vi "YokoGS200 Get Output.vi"(0 "VISA Rsrc":refnum<visa-resource-name>="SR530", 3 "error in (no error)":errorcluster) -> (7 "VISA Rsrc Out":refnum<visa-resource-name>="GPIB0::12::INSTR", 8 "Output State":bool, 10 "error out":errorcluster)   [LabVIEW 2019]
panel:
  out "Octet d'état":bool[](array[boolean])
  out "octet d'état":u16
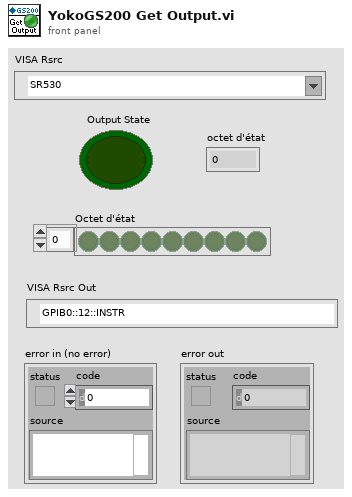
[diagram p1: front panel]
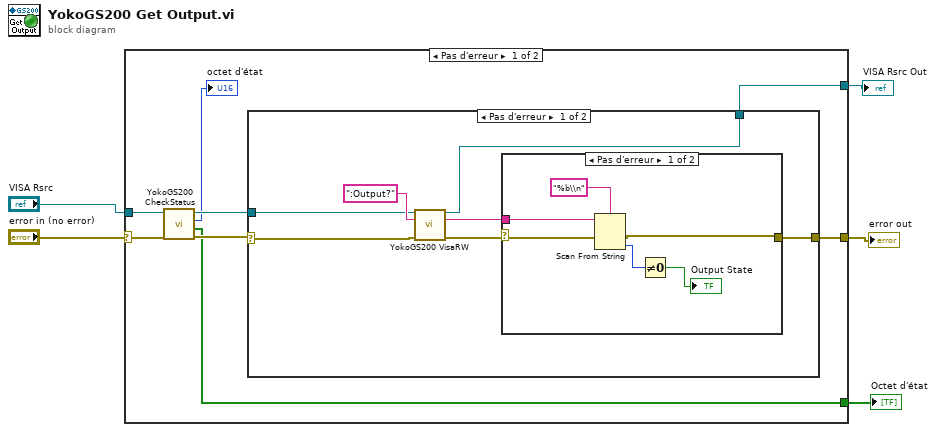
[diagram p0: block diagram]
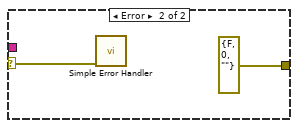
[diagram p2: hidden frame]
diagram:
  n1 = case shown="Pas d'erreur" "error in (no error)" {
    selector: "error in (no error)" -> [w12 w31]
    tunnel: "VISA Rsrc" -> [w11 w32]
    tunnel: [w13 w31] -> w3
    tunnel: [w8 w32] -> w2
    tunnel: [w7 _] -> w1
    frame No Error {
      n2 = call <userlib>:"YokoGS200 CheckStatus.vi"("error in (no error)"=w12, "VISA Rsrc"=w11) -> ("error out"=w10:errorcluster, "Octet d'état"=w7:bool[], "octet d'état"=→"octet d'état":u16, "VISA Rsrc Out"=w9:refnum<visa-resource-name>)  [unwired: 6 in]
      n3 = case shown="Pas d'erreur" w10 {
        selector: w10 -> [w16 w30]
        tunnel: [w19 w30] -> w13
        tunnel: w9 -> [w15 w29]
        tunnel: [w14 w29] -> w8
        frame No Error {
          n4 = call <userlib>:"YokoGS200 VisaRW.vi"("VISA Rsrc"=w15, "ChaineCom"=":Output?" ("initial string"), "error in (no error)"=w16) -> ("VISA Rsrc Out"=w14:refnum<visa-resource-name>, "ChaineRep"=w17:string, "error out"=w18:errorcluster)  [unwired: 8 in, 2 out]
          n5 = case shown="Pas d'erreur" w18 {
            selector: w18 -> [w26 w27]
            tunnel: [w23 errorcluster {"status"=FALSE, "code"=0, "source"=""} ("error IO")] -> w19
            tunnel: w17 -> [w25 _]
            frame No Error {
              n6 = Scan From String(format string="%b\\n", input string=w25, error in=w26) -> (error out=w23:errorcluster, output 1=w22:i32)  [unwired: 2 in, 2 out]
              n7 = Not Equal To 0?(x=w22) -> (x != 0?=→"Output State":bool)
            }
            frame Error {
              n8 = call <vilib>:"Simple Error Handler.vi"("error in (no error)"=w27) -> ()  [unwired: 4 in, 5 out]
            }
          }
        }
        frame Error {
        }
      }
    }
    frame Error {
    }
  }
  "error out" <- w3
  "VISA Rsrc Out" <- w2
  "Octet d'état" <- w1
